vi "LIA Scale Channel Preview.vi"(9 "sample rate":dbl, 10 "scaling factor":dbl, 11 "ai data":i16[](array[numeric])) -> (3 "Waveform":waveform(dbl))   [LabVIEW 2018]
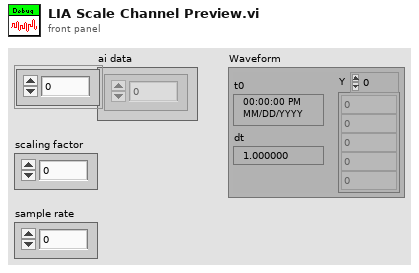
[diagram p1: front panel]
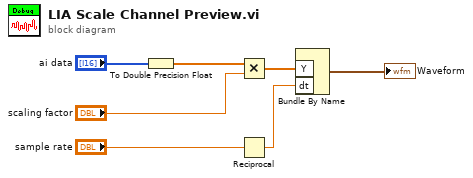
[diagram p0: block diagram]
diagram:
  n1 = To Double Precision Float(number="ai data") -> (double precision float=w2:dbl[])
  n2 = Multiply(x=w2, y="scaling factor") -> (x*y=w4:dbl[])
  n3 = Reciprocal(x="sample rate") -> (1/x=w7:dbl)
  n4 = Bundle By Name("Y"=w4, "dt"=w7) -> (→"Waveform":waveform(dbl))  [unwired: 1 in]
